vi "Service for Authentication.vi"(11 "Shadow Thing":refnum<class "Thing Shadow.lvclass">) -> (2 "Service for Authentication":string)   [LabVIEW 2015, in "NI_AWS_IoT.lvlib" / "Thing Shadow.lvclass"]
uses:
  Thing Shadow.lvclass
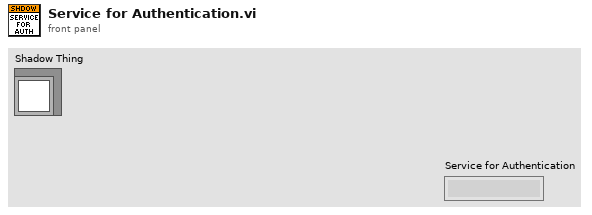
[diagram p1: front panel]
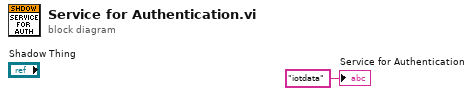
[diagram p0: block diagram]
diagram:
  "Service for Authentication" <- "iotdata" ("Service for Authentication")
